vi "Global_ScorePlayer1.vi"() -> ()   [LabVIEW 2018]
panel:
  in  "ScorePlayer1":u16
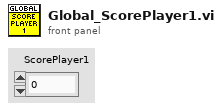
[diagram p1: front panel]
diagram:
